vi "0002_FireAt1015EveryDay.vi"(8 "error in (no error)":errorcluster) -> (0 "error out":errorcluster)   [LabVIEW 2013]
uses:
  <vilib>/addons/_JKI Toolkits/Caraya/classes/Assert/Assert True.vi
  <vilib>/addons/_JKI Toolkits/Caraya/classes/Test/Test.lvclass
  <vilib>/addons/_JKI Toolkits/Caraya/classes/Assert/Assert.lvclass
  source/openCron.lvlib
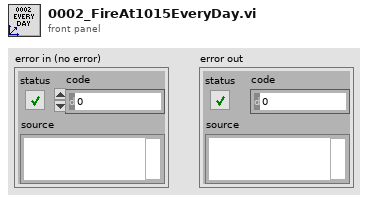
[diagram p1: front panel]
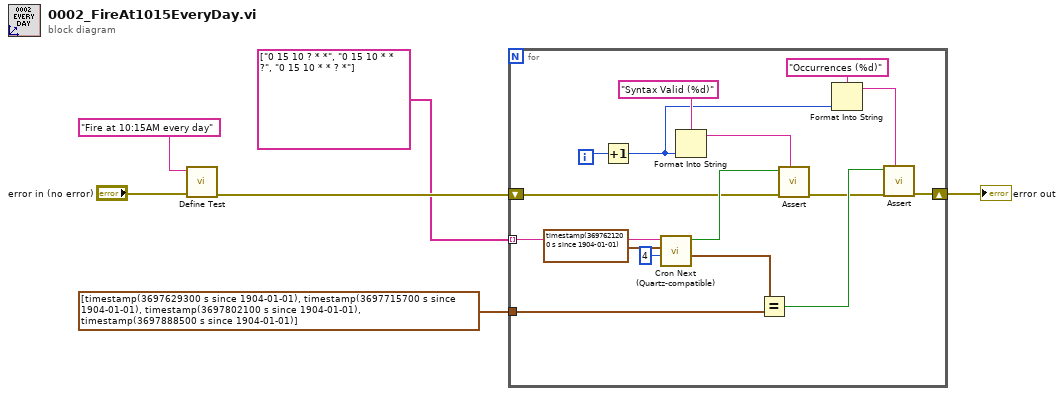
[diagram p0: block diagram]
diagram:
  n1 = call <vilib>:"Define Test.vi"("error in (no error)"="error in (no error)", "Label (VI Title)"="Fire at 10:15AM every day") -> ("error out"=w3:errorcluster)  [unwired: 9 in]
  n2 = for {
    tunnel: timestamp[] [timestamp(3697629300 s since 1904-01-01), timestamp(3697715700 s since 1904-01-01), timestamp(3697802100 s since 1904-01-01), timestamp(3697888500 s since 1904-01-01)] -> [w17]
    tunnel: string[] ["0 15 10 ? * *", "0 15 10 * * ?", "0 15 10 * * ? *"] -> [w13] mode=indexing
    shift-right: [w22] -> w6
    shift-left: w3 -> [w14]
    i -> [w12]
    n3 = Increment(x=w12) -> (x+1=w8:i32)
    n4 = call "Cron Next (Quartz-compatible).vi"("Nb Occurences (min: 1)"=u16 4, "Reference timestamp (Now)"=timestamp(3697621200 s since 1904-01-01) ("y"), "Cron Expression"=w13) -> ("Occurences"=w18:timestamp[], "syntax valid?"=w19:bool)  [unwired: 6 in, 1 out]
    n5 = Format Into String(format string="Syntax Valid (%d)" ("Label (VI Title)"), w8) -> (resulting string=w10:string)  [unwired: 2 in, 1 out]
    n6 = Equal?(x=w18, y=w17) -> (x = y?=w21:bool)
    n7 = call-poly <vilib>:"Assert.vi"("Label"=w10, "error in (no error)"=w14, "True?"=w19) -> ("error out"=w20:errorcluster)  [unwired: 8 in]
    n8 = Format Into String(format string="Occurrences (%d)" ("Label (VI Title)"), w8) -> (resulting string=w7:string)  [unwired: 2 in, 1 out]
    n9 = call-poly <vilib>:"Assert.vi"("Label"=w7, "error in (no error)"=w20, "True?"=w21) -> ("error out"=w22:errorcluster)  [unwired: 8 in]
  }
  "error out" <- w6
